vi "SwerveDrivePoseEst_Kalman_F_Callback.vi"(9 "U":T1, 10 "X":T1, 11 "ExtraPassedData":variant) -> (0 "Error":bool, 3 "Result":T1)   [LabVIEW 2019, in "Trajectory_Library.lvlib"]
doc: "Swerve Drive Pose Estimator, Kalman Filter F function. \n\nThis function returns the U matrix.\n\nInput:\n - ExtraPassedData -- Variant contaiing extra data for the callback For this function the extra data should be empty..\n - X Matrix -- X matrix\n - U Matrix -- U matrix\n\nOutput:\n - Result -- Matrix resulting from calculation\n - Error -- If TRUE an error occured"
uses:
  Trajectory_Library.lvlib
  <vilib>/Analysis/Matrix/Datatypes/RealMatrix.ctl
  <vilib>/Analysis/Matrix/NI_Matrix.lvlib
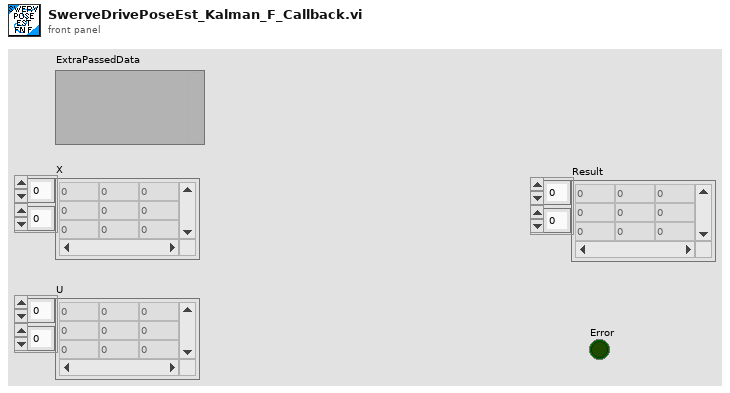
[diagram p1: front panel]
types:
  T1 = typedef "NI_Matrix.lvlib/RealMatrix.ctl" = dbl[][]
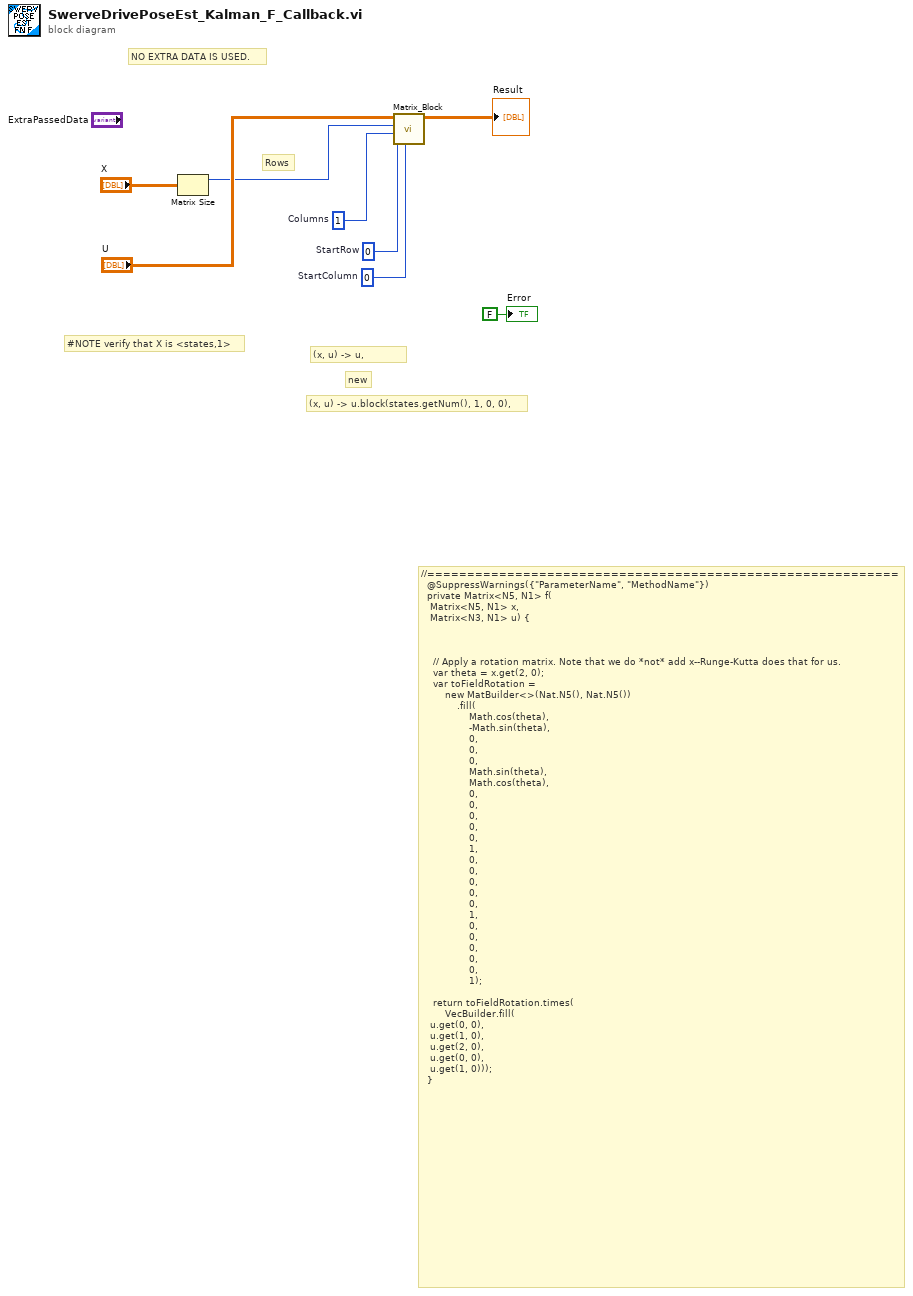
[diagram p0: block diagram]
diagram:
  w4 = 1  # Columns
  w5 = 0  # StartRow
  w6 = 0  # StartColumn
  # "#NOTE verify that X is <states,1>"
  # "new"
  # "Rows"
  # "(x, u) -> u.block(states.getNum(), 1, 0, 0),"
  # "(x, u) -> u,"
  # "NO EXTRA DATA IS USED."
  # "//===========================================================\n  @SuppressWarnings({\"ParameterName\", \"MethodName\"})\n  private Matrix<N5, N1> f(\n\t\t\tMatrix<N5, N1> x, \n\t\t\tMatrix<N3, N1> u) {\n\n\n\n    // Apply a rotation matrix. Note that we do *not* add x--Runge-Kutta does that for us.\n    var theta = x.get(2, 0);\n    var toFieldRotation =\n        new MatBuilder<>(Nat.N5(), Nat.N5())\n            .fill(\n                Math.cos(theta),\n                -Math.sin(theta),\n                0,\n                0,\n                0,\n                Math.sin(theta),\n                Math.cos(theta),\n                0,\n                0,\n                0,\n                0,\n                0,\n                1,\n                0,\n                0,\n                0,\n                0,\n                0,\n                1,\n                0,\n                0,\n                0,\n                0,\n                0,\n                1);\n\n    return toFieldRotation.times(\n        VecBuilder.fill(  \n\t\t\tu.get(0, 0), \n\t\t\tu.get(1, 0), \n\t\t\tu.get(2, 0), \n\t\t\tu.get(0, 0), \n\t\t\tu.get(1, 0)));\n  }"
  n1 = Matrix Size(0:"X") -> (1:w1:i32)  [unwired: 1 out]
  n2 = call "Matrix_Block.vi"("StartColumn"=w6, "StartRow"=w5, "Columns"=w4, "Rows"=w1, "input matrix"="U") -> ("output matrix"=→"Result":T1)  [unwired: 6 in]
  "Error" <- FALSE ("Error")
